vi "GetNodeName.vi"(0 "reference in":refnum<class "ChoiceNode.lvclass">, 5 "error in (no error)":errorcluster) -> (14 "reference out":refnum<class "ChoiceNode.lvclass">, 15 "String":string, 19 "error out":errorcluster)   [LabVIEW 2016, in "ChoiceNode.lvclass"]
uses:
  <resource>/Framework/Providers/Open_GDS/UML/ChoiceNode_class/ChoiceNode.lvclass
  <resource>/Framework/Providers/Open_GDS/UML/MultiLineString_class/MultiLineString.lvclass
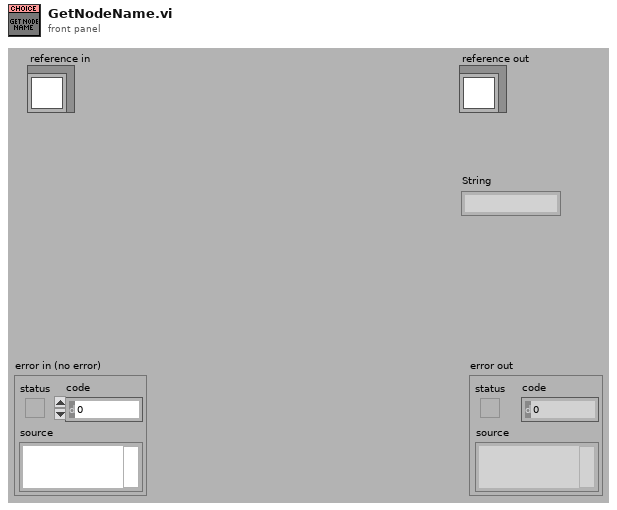
[diagram p1: front panel]
types:
  T1 = typedef "ChoiceNode.lvclass/ObjectAttributes.ctl" = cluster{"Text":refnum<class "MultiLineString.lvclass">, "DEFAULT_WIDTH":i32, "DEFAULT_HEIGHT":i32}
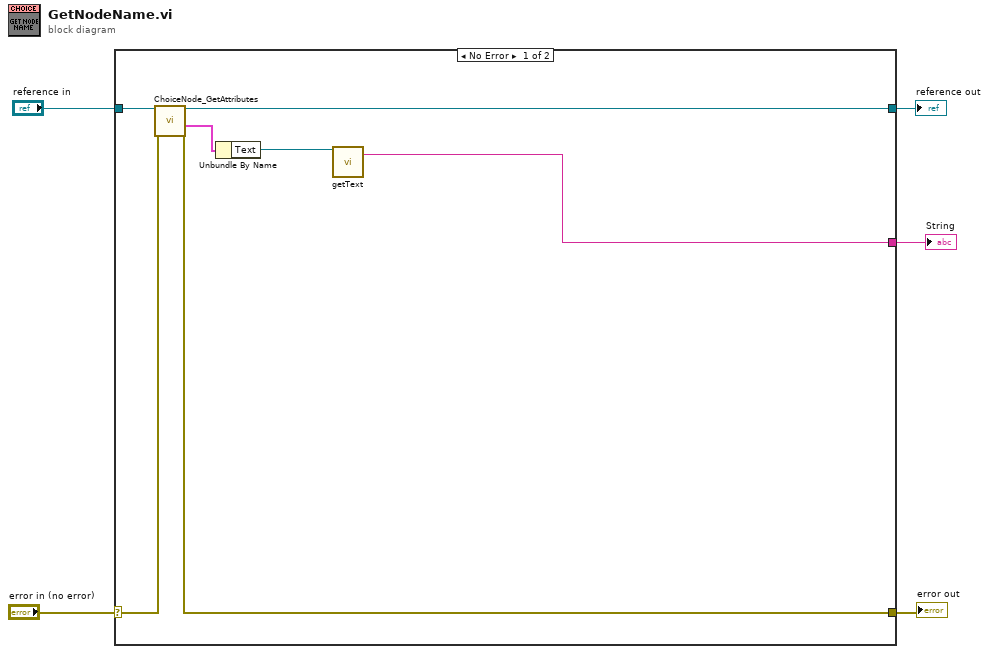
[diagram p0: block diagram]
diagram:
  n1 = case shown="No Error" "error in (no error)" {
    selector: "error in (no error)" -> [w12 w14]
    tunnel: [w11 w14] -> w4
    tunnel: [w9 w13] -> w2
    tunnel: "reference in" -> [w10 w13]
    tunnel: [w7 _] -> w1
    frame No Error {
      n2 = call <resource>:"ChoiceNode_GetAttributes.vi"("reference in"=w10, "error in (no error)"=w12) -> ("reference out"=w9:refnum<class "ChoiceNode.lvclass">, "Data"=w6:T1, "error out"=w11:errorcluster)  [unwired: 14 in, 1 out]
      n3 = Unbundle By Name(w6) -> ("Text"=w8:refnum<class "MultiLineString.lvclass">)
      n4 = call-dynamic "getText.vi"("reference"=w8) -> ("text"=w7:string)  [unwired: 16 in, 2 out]
    }
    frame Error {
    }
  }
  "error out" <- w4
  "reference out" <- w2
  "String" <- w1
